vi "Report Event.vi"(7 "Event Level (Info)":T1, 8 "error in (no error)":errorcluster, 10 "Message":string, 11 "VectoEventBridge in":refnum<class "VectoEventBridge.lvclass">) -> (0 "error out":errorcluster)   [LabVIEW 2020, in "Volatus.lvlib" / "VectoEventBridge.lvclass"]
uses:
  VectoEventBridge.lvclass
  lv-vecto/Vecto/Event Level.ctl
  Event.ctl
  Event Level.ctl
  VectoEventBridge.lvclass/VectoEventBridge.ctl
  MessageQ/MessageQ.lvclass/MessageQ.ctl
  Volatus.lvlib
  MessageQ/MessageQ.lvclass
  lv-vecto/Vecto/Vecto.lvlib
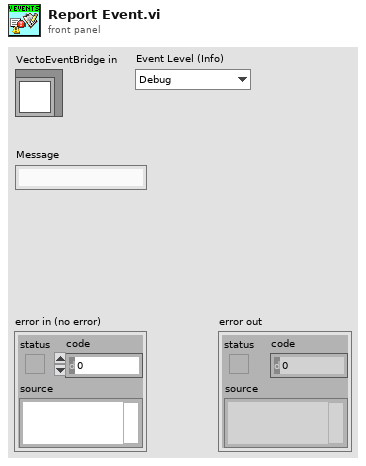
[diagram p1: front panel]
types:
  T1 = typedef "Vecto.lvlib/Event Level.ctl" = enum16{"Debug", "Info", "Warning", "Error"}
  T2 = typedef "Volatus.lvlib/Event.ctl" = cluster{"Time Stamp":timestamp, "Event Level":T3, "Context":string, "Message":string, "Error":errorcluster, "Node":string}
  T3 = typedef "Volatus.lvlib/Event Level.ctl" = enum16{"Debug", "Info", "Warning", "Error"}
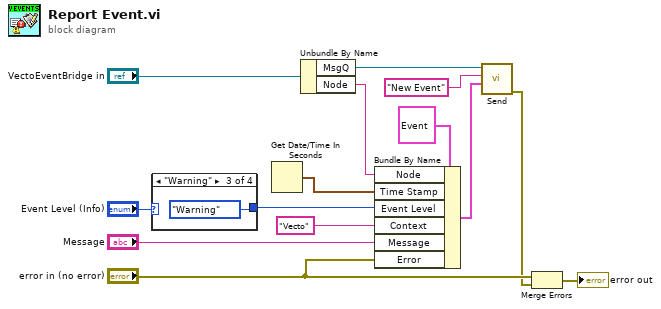
[diagram p0: block diagram]
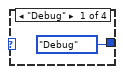
[diagram p2: hidden frame]
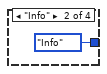
[diagram p3: hidden frame]
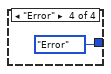
[diagram p4: hidden frame]
diagram:
  n1 = case shown="\"Warning\"" "Event Level (Info)" {
    tunnel: [Event_Level."Debug" ("Event Level") Event_Level."Info" ("Event Level") Event_Level."Warning" ("Event Level") Event_Level."Error" ("Event Level")] -> w9
    frame "Debug" {
    }
    frame "Info" {
    }
    frame "Warning" {
    }
    frame "Error" {
    }
  }
  n2 = Get Date/Time In Seconds() -> (seconds since 1Jan1904=w13:timestamp)
  n3 = Unbundle By Name("VectoEventBridge in") -> ("MsgQ"=w6:refnum<class "MessageQ.lvclass">, "Node"=w1:string)
  n4 = Bundle By Name(cluster=T2 {"Time Stamp"=timestamp(0 s since 1904-01-01), "Event Level"=enum."Info", "Context"="", "Message"="", "Error"={"status"=FALSE, "code"=0, "source"=""}, "Node"=""} ("Event"), "Node"=w1, "Time Stamp"=w13, "Event Level"=w9, "Context"="Vecto", "Message"="Message", "Error"="error in (no error)") -> (w4:T2)
  n5 = call "Send.vi"("Data"=w4, "ID"="New Event", "MessageQ in"=w6) -> ("error out"=w2:errorcluster)  [unwired: 7 in, 1 out]
  n6 = Merge Errors("error in (no error)", w2) -> (→"error out":errorcluster)
